vi "Read.vi"(8 "Error in (no error)":errorcluster, 10 "Byte count":u32, 11 "VISA resource":refnum<visa-resource-name>) -> (0 "Error out":errorcluster, 1 "Return count":u32, 2 "Read buffer":string, 3 "Dup VISA resource":refnum<visa-resource-name>)   [LabVIEW 2010]
doc: "Copyright (c) 2012 Metrolab Technology SA, Plan-les-Ouates, Geneva, Switzerland\nPerforms a VISA Read, and a VISA Clear in case of error.\nThis VI is only used as a sub-VI for Write and Read.vi.\nSee VISA Read for a definition of the parameters."
panel:
  # "Read"
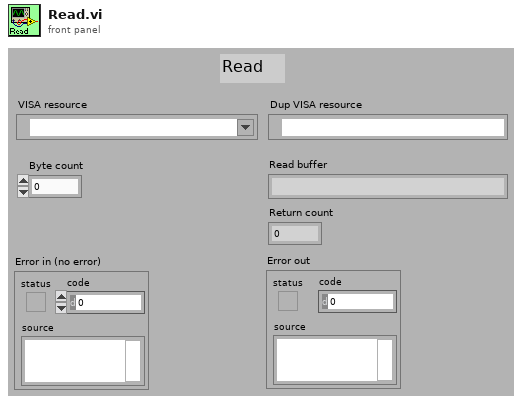
[diagram p1: front panel]
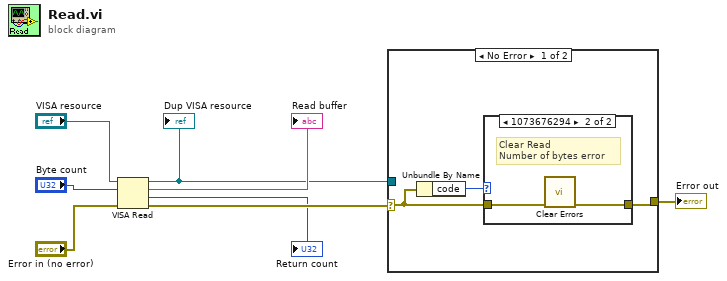
[diagram p0: block diagram]
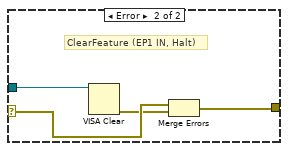
[diagram p3: hidden frame]
diagram:
  n1 = VISA Read(VISA resource name="VISA resource", byte count="Byte count", error in (no error)="Error in (no error)") -> (VISA resource name out=w1:refnum<visa-resource-name>, read buffer=→"Read buffer":string, return count=→"Return count":u32, error out=w4:errorcluster)
  "Dup VISA resource" <- w1
  n2 = case shown="No Error" w4 {
    selector: w4 -> [w10 w18]
    tunnel: w1 -> [_ w16]
    tunnel: [w9 w17] -> w8
    frame No Error {
      n3 = Unbundle By Name(w10) -> ("code"=w11:i32)
      n4 = case shown="1073676294" w11 {
        tunnel: w10 -> [w12 w14]
        tunnel: [w12 w13] -> w9
        frame 0, Default {
        }
        frame 1073676294 {
          # "Clear Read \nNumber of bytes error"
          n5 = call <vilib>:"Clear Errors.vi"("error in (no error)"=w14) -> ("error out"=w13:errorcluster)  [unwired: 6 in]
        }
      }
    }
    frame Error {
      # "ClearFeature (EP1 IN, Halt)"
      n6 = VISA Clear(VISA resource name=w16) -> (error out=w15:errorcluster)  [unwired: 1 in, 1 out]
      n7 = Merge Errors(w18, w15) -> (w17:errorcluster)
    }
  }
  "Error out" <- w8
